vi "PID Control.vi"(4 "umanual":dbl, 5 "dt (sec)":dbl, 6 "manual":i16, 7 "output limit":cluster{"umax":dbl, "umin":dbl}, 8 "Inicialization":T1, 9 "setpoint":dbl, 10 "process variable":dbl, 11 "PID parameters":T2) -> (3 "usat":dbl)   [LabVIEW 2010]
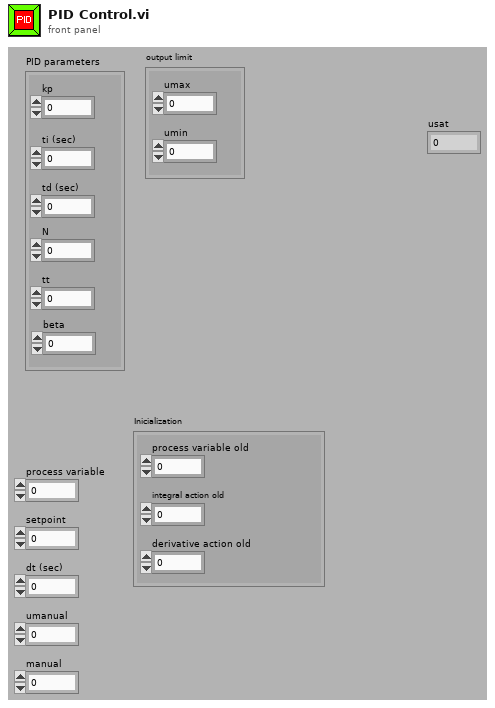
[diagram p1: front panel]
types:
  T1 = cluster{"process variable old":dbl, "integral action old":dbl, "derivative action old":dbl}
  T2 = cluster{"kp":dbl, "ti (sec)":dbl, "td (sec)":dbl, "N":dbl, "tt":dbl, "beta":dbl}
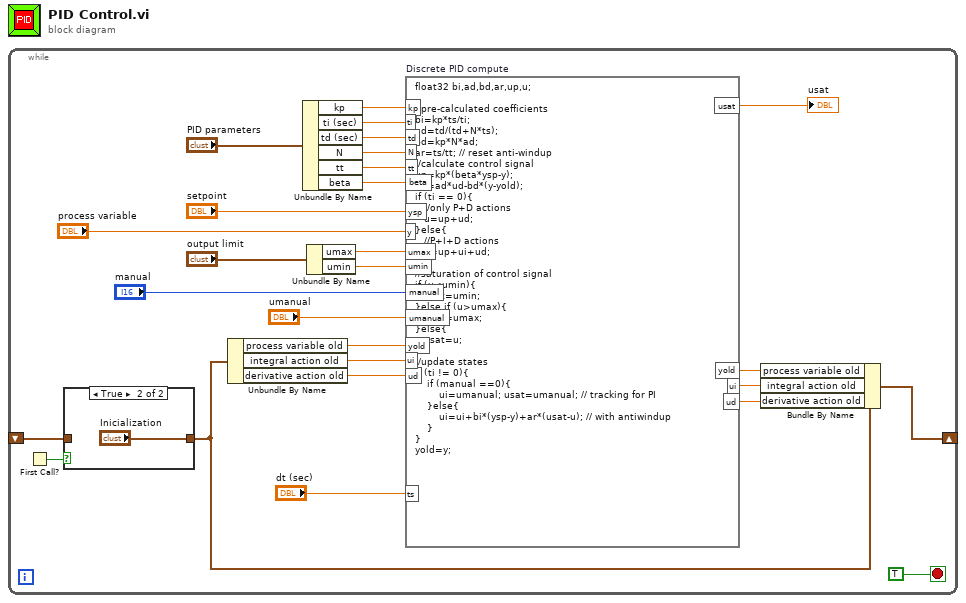
[diagram p0: block diagram]
diagram:
  n1 = while {
    shift-right: [w5] -> _
    shift-left: _ -> [w6]
    stop <- TRUE stop-if-true
    n2 = First Call?() -> (First Call?: T/F=w7:bool)
    n3 = case shown="True" w7 {
      tunnel: [w28 "Inicialization"] -> w13
      tunnel: w6 -> [w28 _]
      frame False {
      }
      frame True {
      }
    }
    n4 = Unbundle By Name(w13) -> ("process variable old"=w19:dbl, "integral action old"=w18:dbl, "derivative action old"=w17:dbl)
    n5 = Unbundle By Name("PID parameters") -> ("kp"=w26:dbl, "ti (sec)"=w25:dbl, "td (sec)"=w24:dbl, "N"=w16:dbl, "tt"=w15:dbl, "beta"=w9:dbl)
    n6 = Unbundle By Name("output limit") -> ("umax"=w4:dbl, "umin"=w3:dbl)
    n7 = formula code="float32 bi,ad,bd,ar,up,u;\n\n//pre-calculated coefficients\nbi=kp*ts/ti;\nad=td/(td+N*ts);\nbd=kp*N*ad;\nar=ts/tt; // reset anti-windup\n//calculate control signal\nup=kp*(beta*ysp-y);\nud=ad*ud-bd*(y-yold);\nif (ti == 0){\n   //only P+D actions\n   u=up+ud;\n}else{\n   //P+I+D actions\n   u=up+ui+ud;\n}\n//saturation of control signal\nif (u<umin){\n   usat=umin;\n}else if (u>umax){\n   usat=umax;\n}else{\n   usat=u;\n}\n//update states\nif (ti != 0){\n    if (manual ==0){\n        ui=umanual; usat=umanual; // tracking for PI\n    }else{\n        ui=ui+bi*(ysp-y)+ar*(usat-u); // with antiwindup\n    }\n}\nyold=y;" "Discrete PID compute"("ts"="dt (sec)", "kp"=w26, "ti"=w25, "td"=w24, "N"=w16, "tt"=w15, "ysp"="setpoint", "y"="process variable", "yold"=w19, "umin"=w3, "umax"=w4, "manual"="manual", "ud"=w17, "ui"=w18, "beta"=w9, "umanual"="umanual") -> ("usat"=→"usat":dbl, "ud"=w10:dbl, "ui"=w11:dbl, "yold"=w12:dbl)
    n8 = Bundle By Name(cluster=w13, "process variable old"=w12, "integral action old"=w11, "derivative action old"=w10) -> (w5:T1)
  }
